vi "SDG X Series Modulated Waveform.vi"() -> ()   [LabVIEW 2015]
doc: "This example shows how to generate a modulated waveform."
uses:
  <instrlib>/SDG X Series/Public/Configure/Configure Modulation (AM).vi
  <instrlib>/SDG X Series/SDG X Series.lvlib
panel:
  in  "VISA resource name":refnum<visa-resource-name>
  in  "Amplitude (1.0 Vpp)":dbl=1.0 format="%#.3f"
  in  "Waveform Function (0: Sine)":u16(ring) items=["Sine", "Square", "Ramp", "DC", "Pulse", "Arb"]
  in  "DC Offset (0.00 V)":dbl
  in  "Frequency (1000 Hz)":dbl=1000.0 format="%#.6g"
  in  "Modulation Frequency (100 Hz)":dbl=100.0
  in  "Modulation Depth (0.0 %)":dbl min=0.0 max=120.0 format="%.1f"
  in  "Modulation Waveform (0: Sine)":u16(ring) items=["Sine", "Square", "Triangle", "UpRamp", "DnRamp", "Noise", "Arb"]
  in  "AM Source (0: Internal)":u16(ring) items=["Internal", "External"]
  in  "Channel (1:Channel 1)":i32(ring)=1 items=["Channel 1"=1, "Channel 2"=2]
  # "(c) 2017 SIGLENT TECHNOLOGIES CO.,LTD. ALL RIGHTS RESERVED."
  # "Modulation Settings"
  # "Carrier Settings"
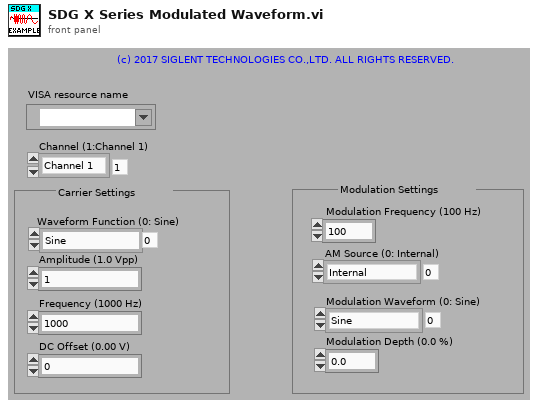
[diagram p1: front panel]
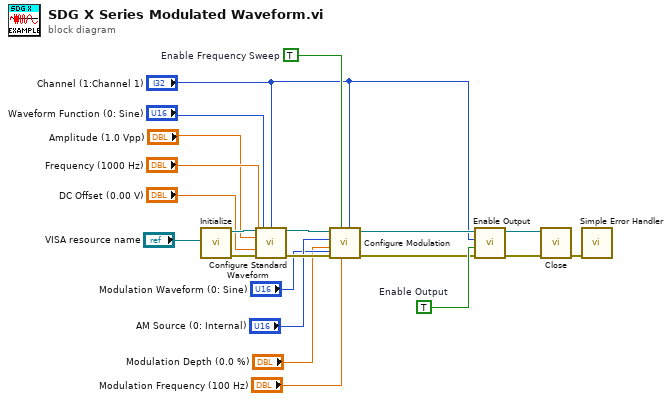
[diagram p0: block diagram]
diagram:
  w15 = TRUE  # Enable Output
  w16 = TRUE  # Enable Frequency Sweep
  n1 = call <instrlib>:"Initialize.vi"("VISA resource name"="VISA resource name") -> ("error out"=w17:errorcluster, "VISA resource name out"=w21:refnum<visa-resource-name>)  [unwired: 9 in]
  n2 = call <instrlib>:"Configure Standard Waveform.vi"("VISA resource name"=w21, "Waveform Function (0: Sine)"="Waveform Function (0: Sine)", "Channel (1:Channel 1)"="Channel (1:Channel 1)", "Amplitude (1.0 Vpp)"="Amplitude (1.0 Vpp)", "Frequency (1000 Hz)"="Frequency (1000 Hz)", "DC Offset (0.00 V)"="DC Offset (0.00 V)", "error in (no error)"=w17) -> ("VISA resource name out"=w18:refnum<visa-resource-name>, "error out"=w19:errorcluster)  [unwired: 7 in]
  n3 = call-poly <instrlib>:"Configure Modulation.vi"("Modulation Waveform (0: Sine)"="Modulation Waveform (0: Sine)", "Channel (1:Channel 1)"="Channel (1:Channel 1)", "Modulation Frequency (100 Hz)"="Modulation Frequency (100 Hz)", "Enable Amplitude Modulation (T:Enable)"=w16, "error in (no error)"=w19, "Modulation Depth (0.0 %)"="Modulation Depth (0.0 %)", "AM Source (0: Internal)"="AM Source (0: Internal)", "VISA resource name"=w18) -> ("error out"=w14:errorcluster, "VISA resource name out"=w13:refnum<visa-resource-name>)  [unwired: 2 in]
  n4 = call <instrlib>:"Enable Output.vi"("error in (no error)"=w14, "Enable Output (T: Enable)"=w15, "Channel (1:Channel 1)"="Channel (1:Channel 1)", "VISA resource name"=w13) -> ("error out"=w6:errorcluster, "VISA resource name out"=w7:refnum<visa-resource-name>)  [unwired: 6 in]
  n5 = call <instrlib>:"Close.vi"("error in (no error)"=w6, "VISA resource name"=w7) -> ("error out"=w20:errorcluster)  [unwired: 9 in]
  n6 = call <vilib>:"Simple Error Handler.vi"("error in (no error)"=w20) -> ()  [unwired: 4 in, 5 out]
